vi "Get Paths and Names.vi"(11 "Stimulus Profiles Base Path Folder":path) -> (2 "Profile Names Out":string[](array[string]), 3 "Paths Out":path[](array[path]))   [LabVIEW 2010]
doc: "This VI takes a base path folder, and returns a list of .et1 & .et2 filenames and full paths."
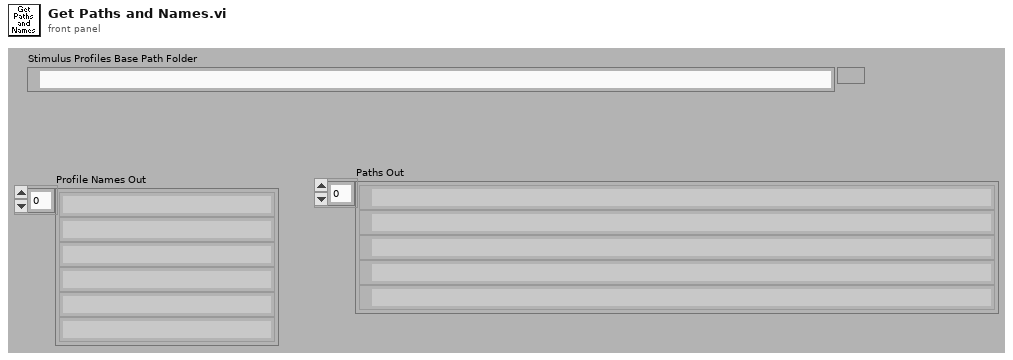
[diagram p1: front panel]
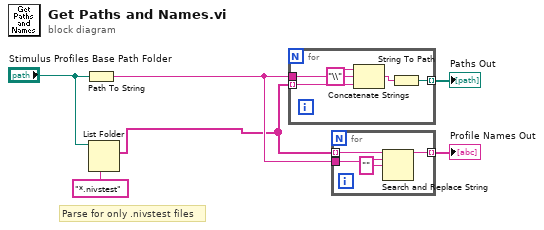
[diagram p0: block diagram]
diagram:
  # "Parse for only .nivstest files"
  n1 = Path To String(path="Stimulus Profiles Base Path Folder") -> (string=w5:string)
  n2 = List Folder(path="Stimulus Profiles Base Path Folder", pattern="*.nivstest") -> (filenames=w1:string[])  [unwired: 2 in, 3 out]
  n3 = for {
    tunnel: w1 -> [w10] mode=indexing
    tunnel: [w11] -> w3 mode=indexing
    tunnel: w5 -> [w7]
    n4 = Concatenate Strings(w7, "\\" ("string"), w10) -> (w9:string)
    n5 = String To Path(string=w9) -> (path=w11:path)
  }
  "Paths Out" <- w3
  n6 = for {
    tunnel: w1 -> [w15] mode=indexing
    tunnel: w5 -> [w14]
    tunnel: [w12] -> w4 mode=indexing
    n7 = Search and Replace String(input string=w15, search string=w14, replace string="" ("replace string (\"\")")) -> (result string=w12:string)  [unwired: 5 in, 3 out]
  }
  "Profile Names Out" <- w4
